vi "ModeMgr.Set Mode.vi"(8 "error in (no error)":errorcluster, 9 "Init":bool, 11 "ModeMgr In":refnum<class "Mode Manager.lvclass">) -> (0 "error out":errorcluster, 1 "Settings":T1[](array[typedef]), 2 "Mode":string, 3 "ModeMgr Out":refnum<class "Mode Manager.lvclass">, 4 "Changed":bool)   [LabVIEW 2018, in "Mode Manager.lvclass"]
uses:
  Mode Manager.lvclass
  ModeMgr.Mode Settings.ctl
  Mode Manager.lvclass/Mode Manager.ctl
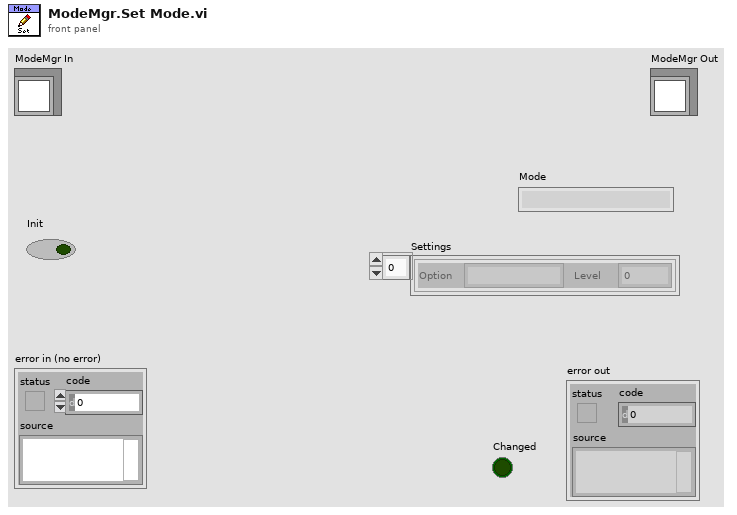
[diagram p1: front panel]
types:
  T1 = typedef "ModeMgr.Mode Settings.ctl" = cluster{"Option":string, "Level":i32}
  T2 = enum32{"invalid app kind", "Development System", "Run Time System", "Student Edition", "Embedded LabVIEW", "Evaluation", "Custom"}
  T3 = cluster{"Changed":bool, "Sel":i32, "Name":string, "Color":string, "Settings":T1[], "Password":string}
  T4 = typedef "ModeMgr.ModeConfig.ctl" = cluster{"Name":string, "Color":string, "Settings":T1[], "Password":string}
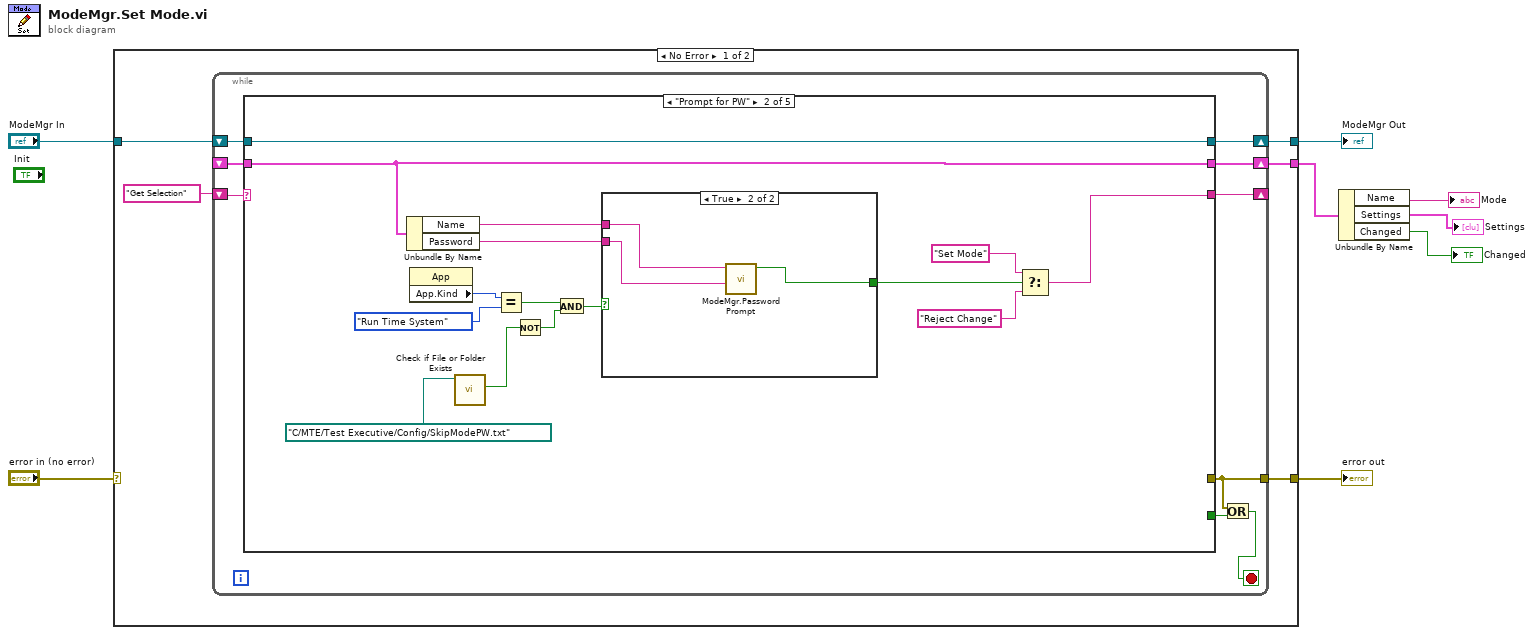
[diagram p0: block diagram]
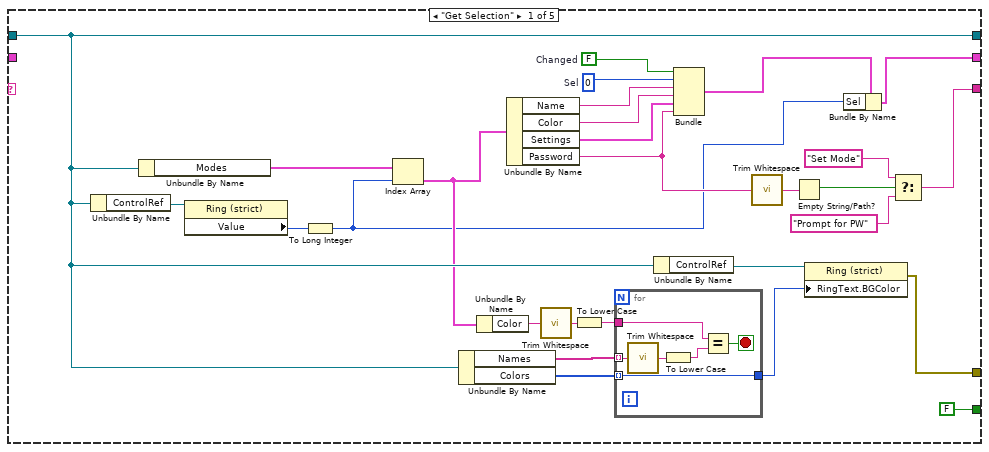
[diagram p2: hidden frame]
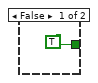
[diagram p3: hidden frame]
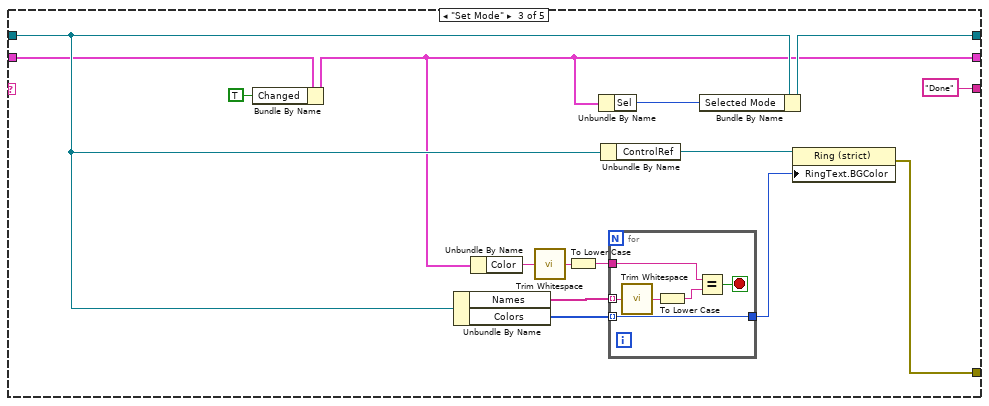
[diagram p4: hidden frame]
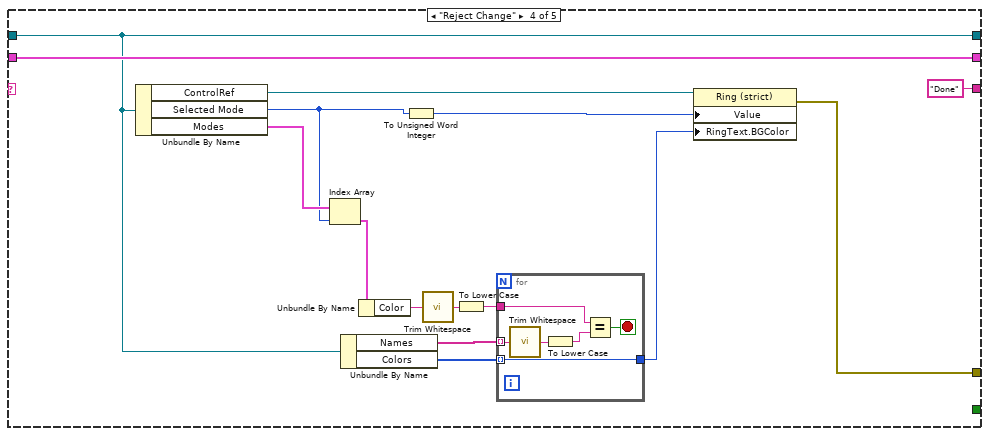
[diagram p5: hidden frame]
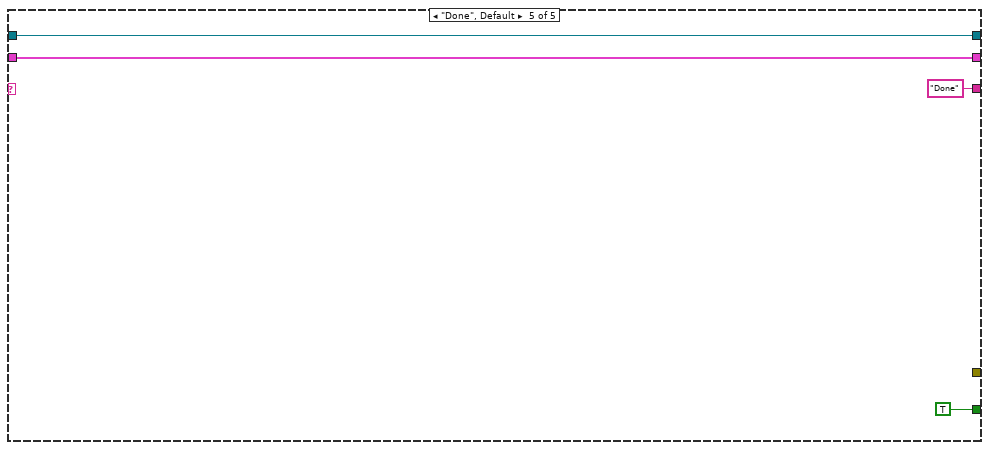
[diagram p6: hidden frame]
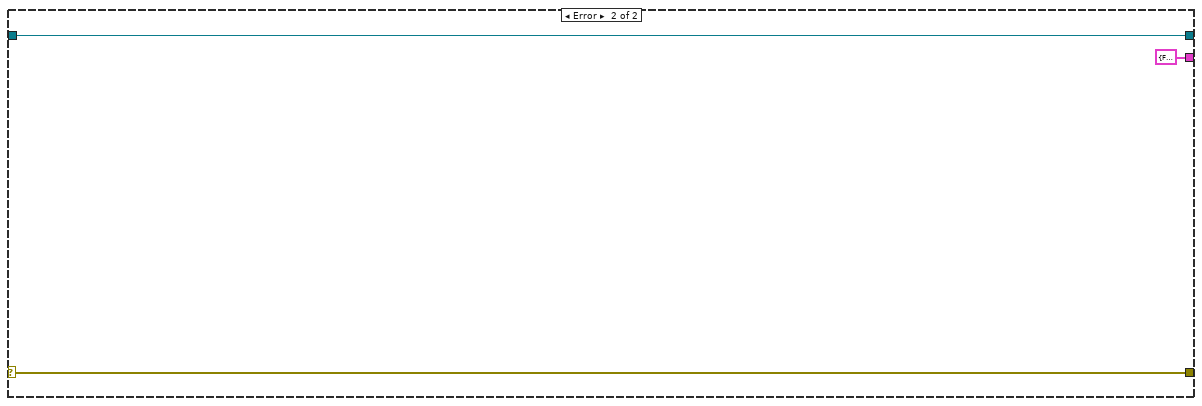
[diagram p7: hidden frame]
diagram:
  n1 = case shown="No Error" "error in (no error)" {
    selector: "error in (no error)" -> [_ w124]
    tunnel: [w13 w124] -> w7
    tunnel: [w12 w123] -> w5
    tunnel: "ModeMgr In" -> [w11 w123]
    tunnel: [w9 T3 {"Changed"=FALSE, "Sel"=0, "Name"="", "Color"="", "Settings"=[], "Password"=""}] -> w4
    frame No Error {
      n2 = while {
        tunnel: [w18] -> w13
        shift-right: [w22] -> w12
        shift-left: w11 -> [w21]
        shift-right: [w14] -> _
        shift-left: "Get Selection" -> [w20]
        shift-right: [w15] -> w9
        shift-left: _ -> [w19]
        stop <- w16 stop-if-true
        n3 = case shown="\"Prompt for PW\"" w20 {
          tunnel: [w28 _ w90 w97 _] -> w18
          tunnel: [w27 w66 w84 w99 w120] -> w22
          tunnel: w21 -> [w27 w66 w83 w99 w120]
          tunnel: w19 -> [_ w64 w78 w111 w121]
          tunnel: [FALSE _ _ _ TRUE] -> w17
          tunnel: [w24 w64 w77 w111 w121] -> w15
          tunnel: [w39 w69 "Done" "Done" "Done"] -> w14
          frame "Get Selection" {
            w36 = FALSE  # Changed
            w46 = 0  # Sel
            n4 = Unbundle By Name(w27) -> ("ControlRef"=w49:refnum<vi>)
            n5 = Unbundle By Name(w27) -> ("Modes"=w50:T4[])
            n6 = property class="Ring (strict)"(reference=w49) -> ("Value"=w48:u16)  [unwired: 1 in, 2 out]
            n7 = To Long Integer(number=w48) -> (32bit integer=w23:i32)
            n8 = Index Array(array=w50, index=w23) -> (element=w26:T4)
            n9 = Unbundle By Name(w27) -> ("Names"=w35:string[], "Colors"=w32:u32[])
            n10 = Unbundle By Name(w26) -> ("Color"=w30:string)
            n11 = Unbundle By Name(w26) -> ("Name"=w45:string, "Color"=w44:string, "Settings"=w38:T1[], "Password"=w37:string)
            n12 = call <vilib>:"Trim Whitespace.vi"("string"=w30) -> ("trimmed string"=w34:string)  [unwired: 1 in]
            n13 = To Lower Case(string=w34) -> (all lower case string=w33:string)
            n14 = for {
              tunnel: w35 -> [w55] mode=indexing
              tunnel: w33 -> [w53]
              tunnel: w32 -> [w51] mode=indexing
              tunnel: [w51] -> w31
              stop <- w52 stop-if-true
              n15 = call <vilib>:"Trim Whitespace.vi"("string"=w55) -> ("trimmed string"=w56:string)  [unwired: 1 in]
              n16 = To Lower Case(string=w56) -> (all lower case string=w54:string)
              n17 = Equal?(x=w53, y=w54) -> (x = y?=w52:bool)
            }
            n18 = Unbundle By Name(w27) -> ("ControlRef"=w29:refnum<vi>)
            n19 = Bundle("Changed"=w36, "Sel"=w46, "Name"=w45, "Color"=w44, "Settings"=w38, "Password"=w37) -> (w25:T3)  [unwired: 1 in]
            n20 = call <vilib>:"Trim Whitespace.vi"("string"=w37) -> ("trimmed string"=w43:string)  [unwired: 1 in]
            n21 = Empty String/Path?(string/path=w43) -> (empty?=w42:bool)
            n22 = property class="Ring (strict)"(reference=w29, "RingText.BGColor"=w31) -> (error out=w28:errorcluster)  [unwired: 1 in, 1 out]
            n23 = Bundle By Name(cluster=w25, "Sel"=w23) -> (w24:T3)
            n24 = Select(t="Set Mode", s=w42, f="Prompt for PW") -> (s? t:f=w39:string)
          }
          frame "Prompt for PW" {
            n25 = Unbundle By Name(w64) -> ("Name"=w68:string, "Password"=w67:string)
            n26 = property class="App"() -> ("App.Kind"=w63:T2)  [unwired: 2 in, 2 out]
            n27 = call <vilib>:"Check if File or Folder Exists.vi"("path"=path "C:/MTE/Test Executive/Config/SkipModePW.txt") -> ("file or folder exists?"=w57:bool)  [unwired: 8 in, 2 out]
            n28 = Equal?(x=w63, y=T2."Run Time System" ("Application:Kind")) -> (x = y?=w59:bool)
            n29 = Not(x=w57) -> (.not. x?=w58:bool)
            n30 = And(x=w59, y=w58) -> (x .and. y?=w61:bool)
            n31 = case shown="True" w61 {
              tunnel: [TRUE w75] -> w65
              tunnel: w68 -> [_ w74]
              tunnel: w67 -> [_ w73]
              frame False {
              }
              frame True {
                n32 = call "ModeMgr.Password Prompt.vi"("Password In"=w73, "Selected Mode"=w74) -> ("Accepted"=w75:bool)  [unwired: 9 in]
              }
            }
            n33 = Select(t="Set Mode", s=w65, f="Reject Change") -> (s? t:f=w69:string)
          }
          frame "Set Mode" {
            n34 = Bundle By Name(cluster=w78, "Changed"=TRUE) -> (w77:T3)
            n35 = Unbundle By Name(w83) -> ("Names"=w89:string[], "Colors"=w86:u32[])
            n36 = Unbundle By Name(w77) -> ("Color"=w82:string)
            n37 = call <vilib>:"Trim Whitespace.vi"("string"=w82) -> ("trimmed string"=w88:string)  [unwired: 1 in]
            n38 = To Lower Case(string=w88) -> (all lower case string=w87:string)
            n39 = Unbundle By Name(w77) -> ("Sel"=w80:i32)
            n40 = Unbundle By Name(w83) -> ("ControlRef"=w81:refnum<vi>)
            n41 = for {
              tunnel: w89 -> [w95] mode=indexing
              tunnel: w87 -> [w93]
              tunnel: w86 -> [w91] mode=indexing
              tunnel: [w91] -> w85
              stop <- w92 stop-if-true
              n42 = call <vilib>:"Trim Whitespace.vi"("string"=w95) -> ("trimmed string"=w96:string)  [unwired: 1 in]
              n43 = To Lower Case(string=w96) -> (all lower case string=w94:string)
              n44 = Equal?(x=w93, y=w94) -> (x = y?=w92:bool)
            }
            n45 = Bundle By Name(cluster=w83, "Selected Mode"=w80) -> (w84:refnum<class "Mode Manager.lvclass">)
            n46 = property class="Ring (strict)"(reference=w81, "RingText.BGColor"=w85) -> (error out=w90:errorcluster)  [unwired: 1 in, 1 out]
          }
          frame "Reject Change" {
            n47 = Unbundle By Name(w99) -> ("ControlRef"=w110:refnum<vi>, "Selected Mode"=w101:i32, "Modes"=w102:T4[])
            n48 = Index Array(array=w102, index=w101) -> (element=w100:T4)
            n49 = Unbundle By Name(w99) -> ("Names"=w107:string[], "Colors"=w104:u32[])
            n50 = Unbundle By Name(w100) -> ("Color"=w103:string)
            n51 = To Unsigned Word Integer(number=w101) -> (unsigned 16bit integer=w109:u16)
            n52 = call <vilib>:"Trim Whitespace.vi"("string"=w103) -> ("trimmed string"=w106:string)  [unwired: 1 in]
            n53 = To Lower Case(string=w106) -> (all lower case string=w105:string)
            n54 = for {
              tunnel: w107 -> [w116] mode=indexing
              tunnel: w105 -> [w114]
              tunnel: w104 -> [w112] mode=indexing
              tunnel: [w112] -> w98
              stop <- w113 stop-if-true
              n55 = call <vilib>:"Trim Whitespace.vi"("string"=w116) -> ("trimmed string"=w117:string)  [unwired: 1 in]
              n56 = To Lower Case(string=w117) -> (all lower case string=w115:string)
              n57 = Equal?(x=w114, y=w115) -> (x = y?=w113:bool)
            }
            n58 = property class="Ring (strict)"(reference=w110, "Value"=w109, "RingText.BGColor"=w98) -> (error out=w97:errorcluster)  [unwired: 1 in, 1 out]
          }
          frame "Done", Default {
          }
        }
        n59 = Or(x=w18, y=w17) -> (x .or. y?=w16:bool)
      }
    }
    frame Error {
    }
  }
  "error out" <- w7
  "ModeMgr Out" <- w5
  n60 = Unbundle By Name(w4) -> ("Name"=→"Mode":string, "Settings"=→"Settings":T1[], "Changed"=→"Changed":bool)
